vi "UI_(06A)_Set_Stop_State.vi"(3 "error in (no error)":errorcluster, 4 "Settings cluster in":T1={"Defaults"={"Default User"=0.0, "VISA Resource Name "=""}, "Recording and saving"={"Researcher name"="", "Name prefix"="", "Data post-processing"={"Filter type"=enum."Savitzky-Golay", "Length"=31, "Order"=3}, "Stop at"=0.0, "\"Stop at\" enabled"=FALSE, "Default save folder path"=path "", "Acquisition FPS"=enum."Max"}, "Geometry"={"Cage diameter, mm"=0, "Starting angle MIDFIELD"=0, "Starting angle BORDER"=0, "Radius, mm CENTER"=0, "Radius, mm MIDFIELD"=0, "N segments MIDFIELD"=0, "N segments BORDER"=0, "R-gap, mm"=0.0, "Bridge swap"=FALSE, "Bridge H. offset"=0.0, "Bridge V. offset"=0.0, "Twisted neck"=FALSE, "Alt. magn. orientation"=FALSE}, "IO parameters"={"IO general config."=0, "IO 1 configuration"=0, "IO 2 configuration"=0, "IO 3 configuration"=0, "IO 4 configuration"=0, "Activate ext. RS-232"=0, "IO inversion config."=0, "Sync capability"=1}, "Stimulus presets array"=[{"Event type"=0, "Dur., s"=0.0, "Stim., s"=0.0, "TTL out N"=1, "Set/Clear"=FALSE, "Stim. has been set"=FALSE}, {"Event type"=0, "Dur., s"=0.0, "Stim., s"=0.0, "TTL out N"=1, "Set/Clear"=FALSE, "Stim. has been set"=FALSE}, {"Event type"=0, "Dur., s"=0.0, "Stim., s"=0.0, "TTL out N"=1, "Set/Clear"=FALSE, "Stim. has been set"=FALSE}, {"Event type"=0, "Dur., s"=0.0, "Stim., s"=0.0, "TTL out N"=1, "Set/Clear"=FALSE, "Stim. has been set"=FALSE}, {"Event type"=0, "Dur., s"=0.0, "Stim., s"=0.0, "TTL out N"=1, "Set/Clear"=FALSE, "Stim. has been set"=FALSE}, {"Event type"=0, "Dur., s"=0.0, "Stim., s"=0.0, "TTL out N"=1, "Set/Clear"=FALSE, "Stim. has been set"=FALSE}, {"Event type"=0, "Dur., s"=0.0, "Stim., s"=0.0, "TTL out N"=1, "Set/Clear"=FALSE, "Stim. has been set"=FALSE}, {"Event type"=0, "Dur., s"=0.0, "Stim., s"=0.0, "TTL out N"=1, "Set/Clear"=FALSE, "Stim. has been set"=FALSE}, {"Event type"=0, "Dur., s"=0.0, "Stim., s"=0.0, "TTL out N"=1, "Set/Clear"=FALSE, "Stim. has been set"=FALSE}, {"Event type"=0, "Dur., s"=0.0, "Stim., s"=0.0, "TTL out N"=1, "Set/Clear"=FALSE, "Stim. has been set"=FALSE}, {"Event type"=0, "Dur., s"=0.0, "Stim., s"=0.0, "TTL out N"=1, "Set/Clear"=FALSE, "Stim. has been set"=FALSE}, {"Event type"=0, "Dur., s"=0.0, "Stim., s"=0.0, "TTL out N"=1, "Set/Clear"=FALSE, "Stim. has been set"=FALSE}, {"Event type"=0, "Dur., s"=0.0, "Stim., s"=0.0, "TTL out N"=1, "Set/Clear"=FALSE, "Stim. has been set"=FALSE}, {"Event type"=0, "Dur., s"=0.0, "Stim., s"=0.0, "TTL out N"=1, "Set/Clear"=FALSE, "Stim. has been set"=FALSE}], "Calibration parameters"={"Timing calibration sw/hw"=1.0, "True FPS"=80.0, "True frame time, s"=80.0, "Disp. calibration info"=[]}, "Settings loaded OK"=FALSE} {"Calibration parameters"."True frame time, s" format="%.10g"; "Calibration parameters"."Disp. calibration info"."Speed, µl per ms" format="%.3g"; "Calibration parameters"."True FPS" format="%.10g"; "Calibration parameters"."Timing calibration sw/hw" format="%.10g"; "Stimulus presets array"."Event type" items=["Stay for N seconds"]; "Stimulus presets array"."TTL out N" items=["1"=1, "2"=2, "1+2"=3]; "Recording and saving"."Data post-processing"."Order" min=3 max=11 step=2; "Recording and saving"."Data post-processing"."Length" min=5 max=301 step=2; "Geometry"."Cage diameter, mm" scale=0.0..340.0}, 5 "All references in":T11) -> (0 "error out":errorcluster, 1 "Settings cluster out":T1={"Defaults"={"Default User"=0.0, "VISA Resource Name "=""}, "Recording and saving"={"Researcher name"="", "Name prefix"="", "Data post-processing"={"Filter type"=enum."Savitzky-Golay", "Length"=31, "Order"=3}, "Stop at"=0.0, "\"Stop at\" enabled"=FALSE, "Default save folder path"=path "", "Acquisition FPS"=enum."Max"}, "Geometry"={"Cage diameter, mm"=0, "Starting angle MIDFIELD"=0, "Starting angle BORDER"=0, "Radius, mm CENTER"=0, "Radius, mm MIDFIELD"=0, "N segments MIDFIELD"=0, "N segments BORDER"=0, "R-gap, mm"=0.0, "Bridge swap"=FALSE, "Bridge H. offset"=0.0, "Bridge V. offset"=0.0, "Twisted neck"=FALSE, "Alt. magn. orientation"=FALSE}, "IO parameters"={"IO general config."=0, "IO 1 configuration"=0, "IO 2 configuration"=0, "IO 3 configuration"=0, "IO 4 configuration"=0, "Activate ext. RS-232"=0, "IO inversion config."=0, "Sync capability"=1}, "Stimulus presets array"=[{"Event type"=0, "Dur., s"=0.0, "Stim., s"=0.0, "TTL out N"=1, "Set/Clear"=FALSE, "Stim. has been set"=FALSE}, {"Event type"=0, "Dur., s"=0.0, "Stim., s"=0.0, "TTL out N"=1, "Set/Clear"=FALSE, "Stim. has been set"=FALSE}, {"Event type"=0, "Dur., s"=0.0, "Stim., s"=0.0, "TTL out N"=1, "Set/Clear"=FALSE, "Stim. has been set"=FALSE}, {"Event type"=0, "Dur., s"=0.0, "Stim., s"=0.0, "TTL out N"=1, "Set/Clear"=FALSE, "Stim. has been set"=FALSE}, {"Event type"=0, "Dur., s"=0.0, "Stim., s"=0.0, "TTL out N"=1, "Set/Clear"=FALSE, "Stim. has been set"=FALSE}, {"Event type"=0, "Dur., s"=0.0, "Stim., s"=0.0, "TTL out N"=1, "Set/Clear"=FALSE, "Stim. has been set"=FALSE}, {"Event type"=0, "Dur., s"=0.0, "Stim., s"=0.0, "TTL out N"=1, "Set/Clear"=FALSE, "Stim. has been set"=FALSE}, {"Event type"=0, "Dur., s"=0.0, "Stim., s"=0.0, "TTL out N"=1, "Set/Clear"=FALSE, "Stim. has been set"=FALSE}, {"Event type"=0, "Dur., s"=0.0, "Stim., s"=0.0, "TTL out N"=1, "Set/Clear"=FALSE, "Stim. has been set"=FALSE}, {"Event type"=0, "Dur., s"=0.0, "Stim., s"=0.0, "TTL out N"=1, "Set/Clear"=FALSE, "Stim. has been set"=FALSE}, {"Event type"=0, "Dur., s"=0.0, "Stim., s"=0.0, "TTL out N"=1, "Set/Clear"=FALSE, "Stim. has been set"=FALSE}, {"Event type"=0, "Dur., s"=0.0, "Stim., s"=0.0, "TTL out N"=1, "Set/Clear"=FALSE, "Stim. has been set"=FALSE}, {"Event type"=0, "Dur., s"=0.0, "Stim., s"=0.0, "TTL out N"=1, "Set/Clear"=FALSE, "Stim. has been set"=FALSE}, {"Event type"=0, "Dur., s"=0.0, "Stim., s"=0.0, "TTL out N"=1, "Set/Clear"=FALSE, "Stim. has been set"=FALSE}], "Calibration parameters"={"Timing calibration sw/hw"=1.0, "True FPS"=80.0, "True frame time, s"=80.0, "Disp. calibration info"=[]}, "Settings loaded OK"=FALSE} {"Calibration parameters"."True frame time, s" format="%.10g"; "Calibration parameters"."Disp. calibration info"."Speed, µl per ms" format="%.3g"; "Calibration parameters"."True FPS" format="%.10g"; "Calibration parameters"."Timing calibration sw/hw" format="%.10g"; "Stimulus presets array"."Event type" items=["Stay for N seconds"]; "Stimulus presets array"."TTL out N" items=["1"=1, "2"=2, "1+2"=3]; "Recording and saving"."Data post-processing"."Order" min=3 max=11 step=2; "Recording and saving"."Data post-processing"."Length" min=5 max=301 step=2; "Geometry"."Cage diameter, mm" scale=0.0..340.0}, 2 "All references out":T11)   [LabVIEW 2018, in "Tracker.lvlib"]
uses:
  Tracker.lvlib
  Controls/CTL_All_References.ctl
  Controls/CTL_Controls_References.ctl
  Controls/CTL_Indicators_References.ctl
  Controls/CTL_Panes_and_VIs_References.ctl
  Controls/CTL_Histogram_Properties.ctl
  <vilib>/Utility/miscctls.llb/LVRangeTypeDef.ctl
  Controls/CTL_Settings_cluster.ctl
  Controls/CTL_Filter_selector.ctl
  Controls/CTL_Acquisition_speed_selector.ctl
  Controls/CTL_Segmented_plot_parameters.ctl
  Controls/CTL_IO_params_cluster.ctl
  Controls/CTL_Single_stimulus_setting.ctl
  Controls/CTL_Calibration_parameters.ctl
  Controls/CTL_Dispenser_calibration_info.ctl
  <vilib>/Utility/error.llb/Error Cluster From Error Code.vi
  <vilib>/ErrorRing/Error Ring.xnode
panel:
  in  "Histogram initialization cluster":T9={"X Scale.Range"={"Minimum"=0.0, "Maximum"=13.0, "Increment"=1.0, "Minor Increment"=1.0, "Start"=0.0}, "Caption.Text"="Zone preference (normalized)", "X Scale.Offset and Multiplier:Multiplier"=1.0, "X Scale.Offset and Multiplier:Offset"=0.0, "X Scale.Scale Fit"=2, "X Scale.Display Format:Precision"=0, "Y Scale.Mapping Mode"=0, "Zones preference empty initialized array"=[0, 0, 0, 0, 0, 0, 0, 0, 0, 0, 0, 0, 0, 0], "Plot.Fill/Point Color"=15790320}
  out "Panes references":T14
  out "Controls references params":string[][](array[string])
  out "Indicators references params":string[][](array[string])
  out "Indicators references":T13
  out "Controls references":T12
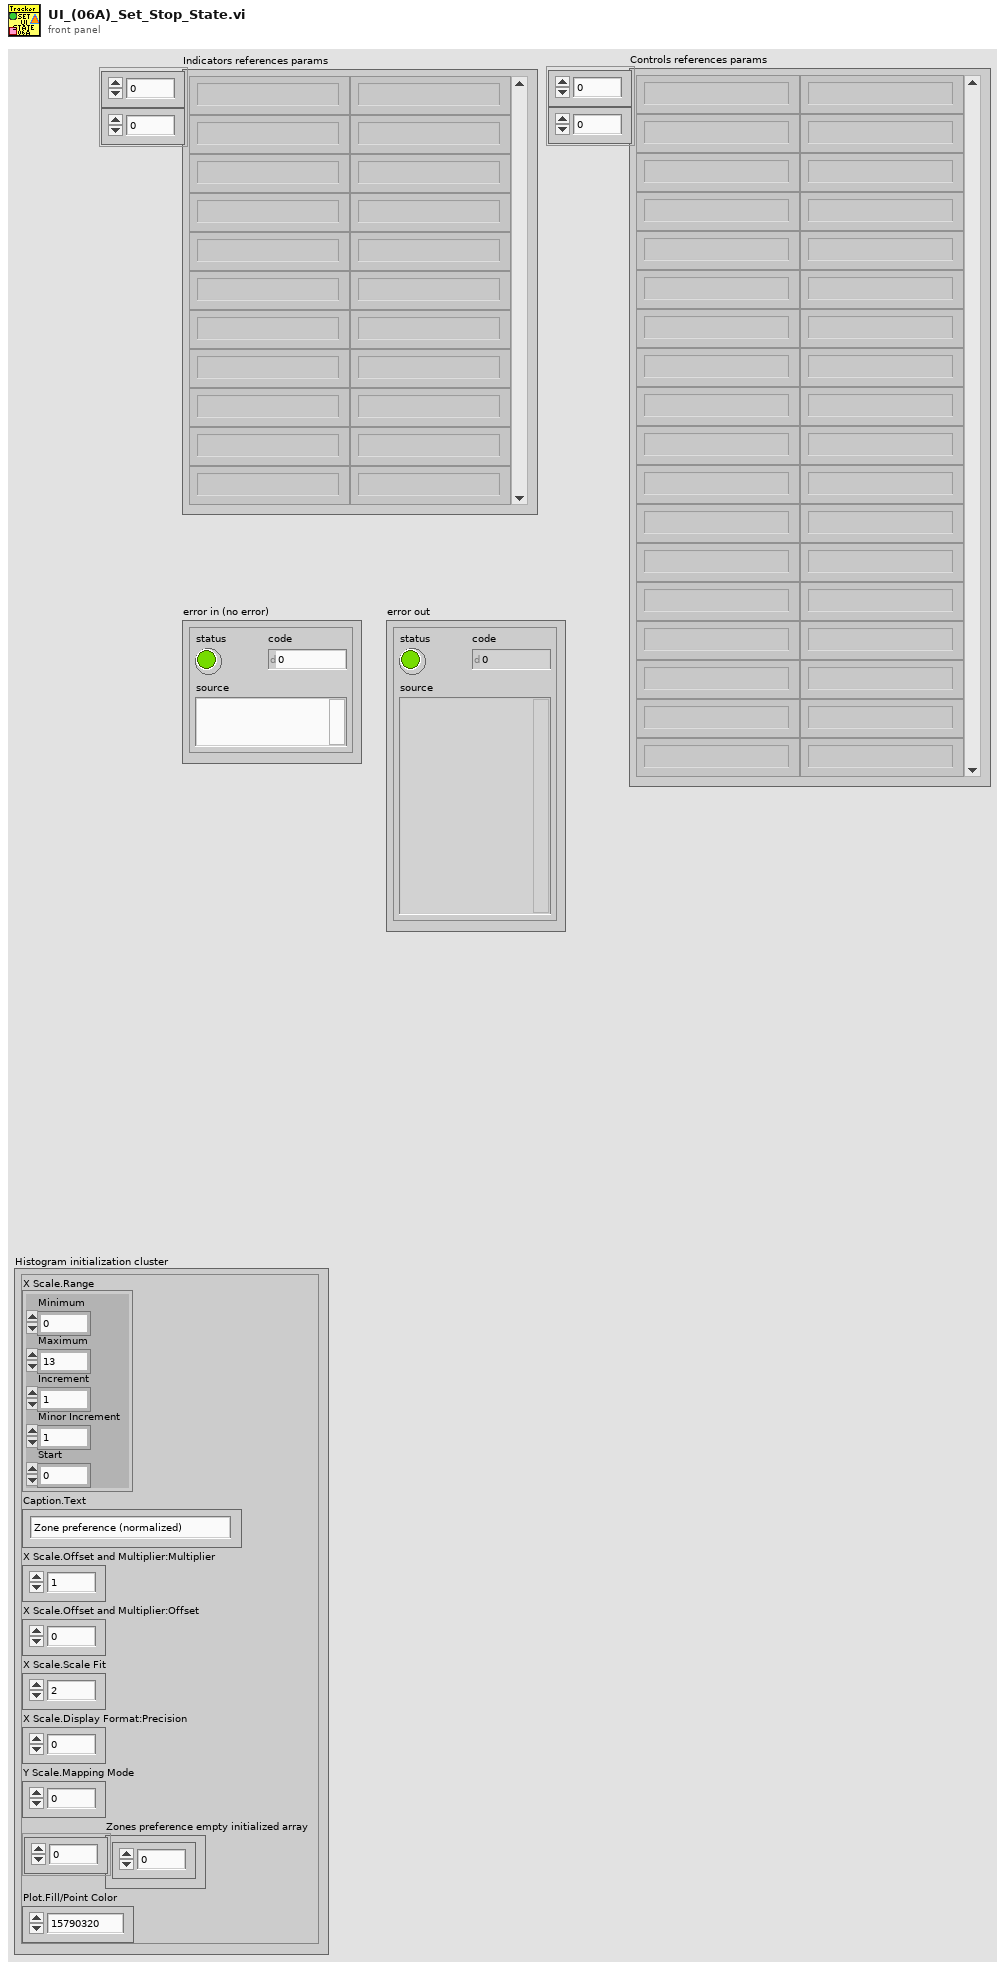
[diagram p1: front panel]
types:
  T1 = typedef "Tracker.lvlib/CTL_Settings_cluster.ctl" = cluster{"Defaults":cluster{"Default User":dbl, "VISA Resource Name ":string}, "Recording and saving":cluster{"Researcher name":string, "Name prefix":string, "Data post-processing":T2, "Stop at":dbl, "\"Stop at\" enabled":bool, "Default save folder path":path, "Acquisition FPS":T3}, "Geometry":T4, "IO parameters":T5, "Stimulus presets array":T6[], "Calibration parameters":T7, "Settings loaded OK":bool}
  T2 = typedef "Tracker.lvlib/CTL_Filter_selector.ctl" = cluster{"Filter type":enum16{"None", "Savitzky-Golay"}, "Length":i32, "Order":i32}
  T3 = typedef "Tracker.lvlib/CTL_Acquisition_speed_selector.ctl" = enum16{"Max", "Optimal", "Eco"}
  T4 = typedef "Tracker.lvlib/CTL_Segmented_plot_parameters.ctl" = cluster{"Cage diameter, mm":u16, "Starting angle MIDFIELD":i16, "Starting angle BORDER":i16, "Radius, mm CENTER":u16, "Radius, mm MIDFIELD":u16, "N segments MIDFIELD":u8, "N segments BORDER":u8, "R-gap, mm":sgl, "Bridge swap":bool, "Bridge H. offset":sgl, "Bridge V. offset":sgl, "Twisted neck":bool, "Alt. magn. orientation":bool}
  T5 = typedef "Tracker.lvlib/CTL_IO_params_cluster.ctl" = cluster{"IO general config.":u16, "IO 1 configuration":u16, "IO 2 configuration":u16, "IO 3 configuration":u16, "IO 4 configuration":u16, "Activate ext. RS-232":u16, "IO inversion config.":u16, "Sync capability":u8}
  T6 = typedef "Tracker.lvlib/CTL_Single_stimulus_setting.ctl" = cluster{"Event type":u16, "Dur., s":sgl, "Stim., s":sgl, "TTL out N":u16, "Set/Clear":bool, "Stim. has been set":bool}
  T7 = typedef "Tracker.lvlib/CTL_Calibration_parameters.ctl" = cluster{"Timing calibration sw/hw":dbl, "True FPS":dbl, "True frame time, s":dbl, "Disp. calibration info":T8}
  T8 = typedef "Tracker.lvlib/CTL_Dispenser_calibration_info.ctl" = cluster{"Channel":u8, "Speed, µl per ms":dbl}[]
  T9 = typedef "Tracker.lvlib/CTL_Histogram_Properties.ctl" = cluster{"X Scale.Range":T10, "Caption.Text":string, "X Scale.Offset and Multiplier:Multiplier":dbl, "X Scale.Offset and Multiplier:Offset":dbl, "X Scale.Scale Fit":u8, "X Scale.Display Format:Precision":u8, "Y Scale.Mapping Mode":u8, "Zones preference empty initialized array":i32[], "Plot.Fill/Point Color":u32}
  T10 = typedef "LVRangeTypeDef.ctl" = cluster{"Minimum":dbl, "Maximum":dbl, "Increment":dbl, "Minor Increment":dbl, "Start":dbl}
  T11 = typedef "Tracker.lvlib/CTL_All_References.ctl" = cluster{"Controls references":T12, "Indicators references":T13, "Service references":T14}
  T12 = typedef "Tracker.lvlib/CTL_Controls_References.ctl" = cluster{"Check HW connection":refnum<vi>, "Start Tracking button":refnum<vi>, "Reset zones":refnum<vi>, "Reset stimuli":refnum<vi>, "Record/Stop":refnum<vi>, "Reset barplot":refnum<vi>, "Multiplyer of chart RX":refnum<vi>, "Show zones":refnum<vi>, "Show magnets":refnum<vi>, "Show heatmap":refnum<vi>, "Show full track":refnum<vi>, "Open File":refnum<vi>, "Play/Pause":refnum<vi>, "Trace, s":refnum<vi>, "Playback speed":refnum<vi>, "Timeline":refnum<vi>, "By Zone stim. setup":refnum<vi>, "Set, Rec and Analyse Tab":refnum<vi>, "Cage radial segmentation":refnum<vi>, "Set IO config":refnum<vi>, "Rainbow (time)":refnum<vi>, "Rainbow (speed)":refnum<vi>}
  T13 = typedef "Tracker.lvlib/CTL_Indicators_References.ctl" = cluster{"HW info":refnum<vi>, "Port":refnum<vi>, "Ready":refnum<vi>, "IO status indicator":refnum<vi>, "Current Time":refnum<vi>, "Record timestamp":refnum<vi>, "Mouse speed":refnum<vi>, "Mouse speed, mm/s":refnum<vi>, "Running, perc. of time":refnum<vi>, "Histograms":refnum<vi>, "Cage size":refnum<vi>}
  T14 = typedef "Tracker.lvlib/CTL_Panes_and_VIs_References.ctl" = cluster{"Pane":refnum<vi>, "This VI":refnum<vi>, "Menu":refnum<k9>}
  T15 = enum8{"Enabled", "Disabled", "Disabled and Grayed Out"}
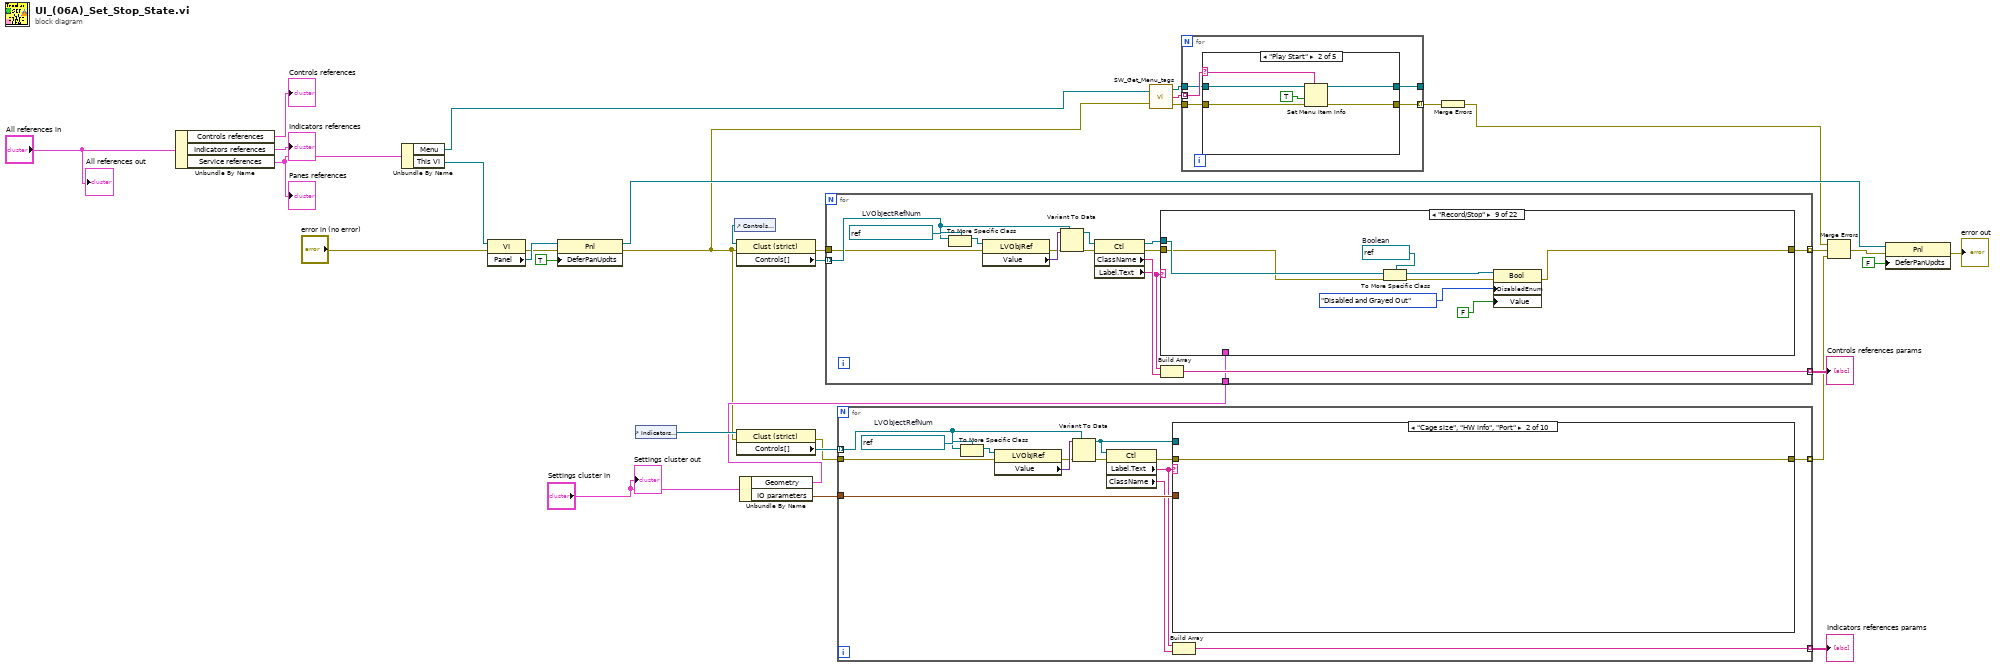
[diagram p0: block diagram]
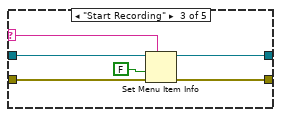
[diagram p3: hidden frame]
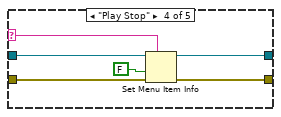
[diagram p4: hidden frame]
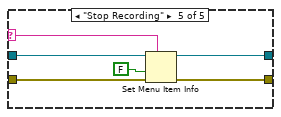
[diagram p5: hidden frame]
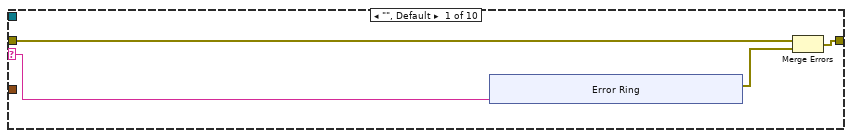
[diagram p6: hidden frame]
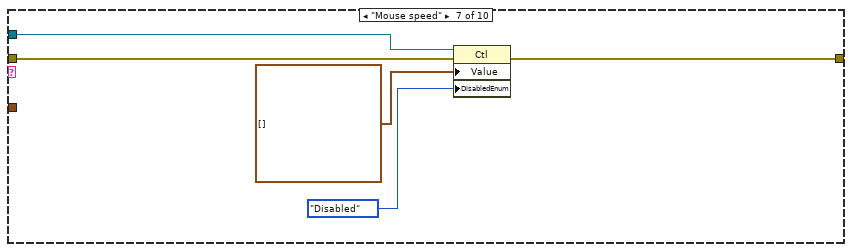
[diagram p11: hidden frame]
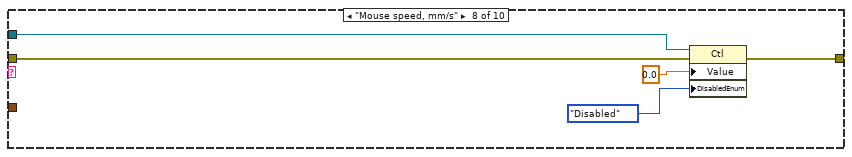
[diagram p12: hidden frame]
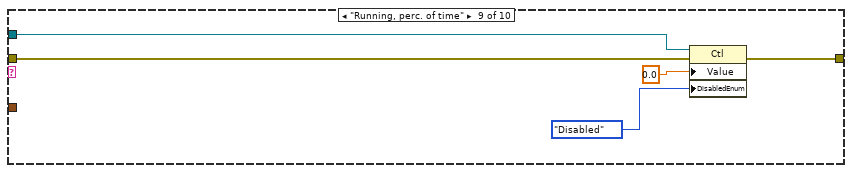
[diagram p13: hidden frame]
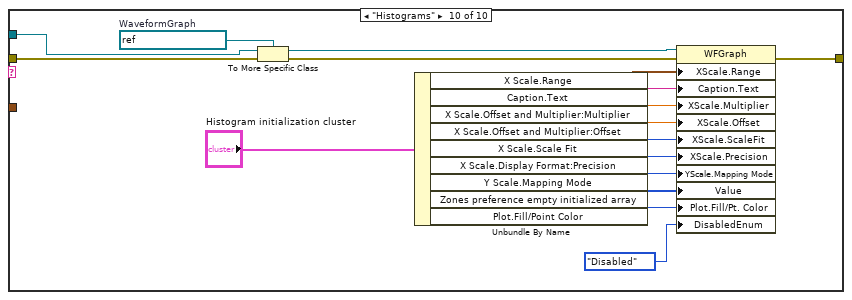
[diagram p14: hidden frame]
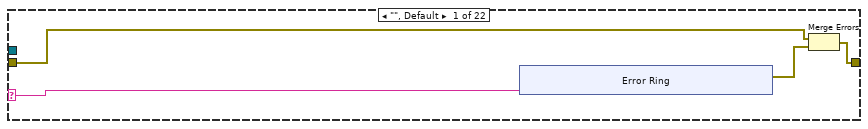
[diagram p15: hidden frame]
diagram:
  n1 = Unbundle By Name("All references in") -> ("Controls references"=→"Controls references":T12, "Indicators references"=→"Indicators references":T13, "Service references"=w24:T14)
  "Panes references" <- w24
  n2 = Unbundle By Name(w24) -> ("Menu"=w3:refnum<k9>, "This VI"=w21:refnum<vi>)
  n3 = property class="VI"(reference=w21, error in="error in (no error)") -> (error out=w14:errorcluster, "Panel"=w23:refnum<vi>)  [unwired: 1 out]
  n4 = property class="Pnl"(reference=w23, error in=w14, "DeferPanUpdts"=TRUE ("Defer Panel Updates")) -> (reference out=w15:refnum<vi>, error out=w2:errorcluster)
  n5 = control-ref of="Indicators references"() -> (w27:refnum<vi>)
  n6 = control-ref of="Controls references"() -> (w29:refnum<vi>)
  n7 = property class="Clust (strict)"(reference=w29, error in=w2) -> (error out=w20:errorcluster, "Controls[]"=w30:refnum<vi>[])  [unwired: 1 out]
  n8 = property class="Clust (strict)"(reference=w27, error in=w2) -> (error out=w19:errorcluster, "Controls[]"=w28:refnum<vi>[])  [unwired: 1 out]
  n9 = Unbundle By Name("Settings cluster in") -> ("Geometry"=w8:T4, "IO parameters"=w10:T5)
  n10 = for {
    tunnel: w30 -> [w45] mode=indexing
    tunnel: [w42] -> w25 mode=indexing
    tunnel: w20 -> [w41]
    tunnel: [w37] -> w12 mode=indexing
    tunnel: w8 -> [w34]
    w47 = refnum<vi> refnum  # LVObjectRefNum
    n11 = To More Specific Class(target class=w47, reference=w45) -> (specific class reference=w48:refnum<vi>)  [unwired: 1 in, 1 out]
    n12 = property class="LVObjRef"(reference=w48, error in=w41) -> (error out=w40:errorcluster, "Value"=w46:variant)  [unwired: 1 out]
    n13 = Variant To Data(error in=w40, type=w45, Variant=w46) -> (data=w44:refnum<vi>, error out=w39:errorcluster)
    n14 = property class="Ctl"(reference=w44, error in=w39) -> (reference out=w35:refnum<vi>, error out=w36:errorcluster, "ClassName"=w43:string, "Label.Text"=w38:string)
    n15 = case shown="\"Record/Stop\"" w38 {
      selector: w38 -> [w49 _ _ _ _ _ _ _ _ _ _ _ _ _ _ _ _ _ _ _ _ _]
      tunnel: [w51 w60 w61 w62 w63 w64 w65 w66 w67 w77 w85 w93 w99 w100 w109 w117 w123 w125 w134 w142 w150 w156] -> w37
      tunnel: w36 -> [w52 w60 w61 w62 w63 w64 w65 w66 w68 w79 w87 w95 w99 w102 w111 w119 w123 w126 w136 w144 w152 w156]
      tunnel: w35 -> [_ _ _ _ _ _ _ _ w69 w82 w90 w98 _ w101 w114 w122 _ w127 w139 w147 w155 _]
      tunnel: w34 -> [_ _ _ _ _ _ _ _ _ _ _ _ _ _ _ _ _ _ _ _ _ _]
      frame "", Default {
        n16 = xnode "Error Ring"("parameter 0"=w49) -> ("error out"=w50:errorcluster)
        n17 = Merge Errors(w52, w50) -> (w51:errorcluster)
      }
      frame "Cage radial segmentation" {
      }
      frame "Set/Rec and Analyse Tab" {
      }
      frame "Check HW connection" {
      }
      frame "Save settings" {
      }
      frame "Set IO config" {
      }
      frame "Reset zones" {
      }
      frame "Reset stimuli" {
      }
      frame "Record/Stop" {
        w70 = refnum<vi> refnum  # Boolean
        n18 = To More Specific Class(target class=w70, reference=w69, error in=w68) -> (specific class reference=w74:refnum<vi>, error out=w73:errorcluster)
        n19 = property class="Bool"(reference=w74, error in=w73, "DisabledEnum"=T15."Disabled and Grayed Out" ("Disabled"), "Value"=FALSE) -> (error out=w67:errorcluster)  [unwired: 1 out]
      }
      frame "Reset barplot" {
        w81 = refnum<vi> refnum  # Boolean
        n20 = To More Specific Class(target class=w81, reference=w82, error in=w79) -> (specific class reference=w80:refnum<vi>, error out=w78:errorcluster)
        n21 = property class="Bool"(reference=w80, error in=w78, "Value"=FALSE, "DisabledEnum"=T15."Enabled" ("Disabled")) -> (error out=w77:errorcluster)  [unwired: 1 out]
      }
      frame "Multiplyer of chart RX" {
        w89 = refnum<vi> refnum  # Slide
        n22 = To More Specific Class(target class=w89, reference=w90, error in=w87) -> (specific class reference=w88:refnum<vi>, error out=w86:errorcluster)
        n23 = property class="Slide"(reference=w88, error in=w86, "Value"=u8 1, "DisabledEnum"=T15."Enabled" ("Disabled")) -> (error out=w85:errorcluster)  [unwired: 1 out]
      }
      frame "Show zones" {
        w97 = refnum<vi> refnum  # Boolean
        n24 = To More Specific Class(target class=w97, reference=w98, error in=w95) -> (specific class reference=w96:refnum<vi>, error out=w94:errorcluster)
        n25 = property class="Bool"(reference=w96, error in=w94, "Value"=TRUE, "DisabledEnum"=T15."Enabled" ("Disabled")) -> (error out=w93:errorcluster)  [unwired: 1 out]
      }
      frame "Show magnets" {
      }
      frame "Rainbow (speed)", "Rainbow (time)" {
        w103 = refnum<vi> refnum  # Boolean
        n26 = To More Specific Class(target class=w103, reference=w101, error in=w102) -> (specific class reference=w105:refnum<vi>, error out=w106:errorcluster)
        n27 = property class="Bool"(reference=w105, error in=w106, "DisabledEnum"=T15."Enabled" ("Disabled")) -> (error out=w100:errorcluster)  [unwired: 1 out]
      }
      frame "Show heatmap" {
        w113 = refnum<vi> refnum  # Boolean
        n28 = To More Specific Class(target class=w113, reference=w114, error in=w111) -> (specific class reference=w112:refnum<vi>, error out=w110:errorcluster)
        n29 = property class="Bool"(reference=w112, error in=w110, "Value"=FALSE, "DisabledEnum"=T15."Disabled and Grayed Out" ("Disabled")) -> (error out=w109:errorcluster)  [unwired: 1 out]
      }
      frame "Show full track" {
        w121 = refnum<vi> refnum  # Boolean
        n30 = To More Specific Class(target class=w121, reference=w122, error in=w119) -> (specific class reference=w120:refnum<vi>, error out=w118:errorcluster)
        n31 = property class="Bool"(reference=w120, error in=w118, "Value"=FALSE, "DisabledEnum"=T15."Disabled and Grayed Out" ("Disabled")) -> (error out=w117:errorcluster)  [unwired: 1 out]
      }
      frame "Open File" {
      }
      frame "Play/Pause" {
        w128 = refnum<vi> refnum  # Boolean
        n32 = To More Specific Class(target class=w128, reference=w127, error in=w126) -> (specific class reference=w131:refnum<vi>, error out=w130:errorcluster)
        n33 = property class="Bool"(reference=w131, error in=w130, "DisabledEnum"=T15."Enabled" ("Disabled"), "Value"=FALSE) -> (error out=w125:errorcluster)  [unwired: 1 out]
      }
      frame "Trace, s" {
        w138 = refnum<vi> refnum  # Slide
        n34 = To More Specific Class(target class=w138, reference=w139, error in=w136) -> (specific class reference=w137:refnum<vi>, error out=w135:errorcluster)
        n35 = property class="Slide"(reference=w137, error in=w135, "Value"=u8 5, "DisabledEnum"=T15."Enabled" ("Disabled")) -> (error out=w134:errorcluster)  [unwired: 1 out]
      }
      frame "Playback speed" {
        w146 = refnum<vi> refnum  # Ring
        n36 = To More Specific Class(target class=w146, reference=w147, error in=w144) -> (specific class reference=w145:refnum<vi>, error out=w143:errorcluster)
        n37 = property class="Ring"(reference=w145, error in=w143, "Value"=u8 3, "DisabledEnum"=T15."Disabled and Grayed Out" ("Disabled")) -> (error out=w142:errorcluster)  [unwired: 1 out]
      }
      frame "Timeline" {
        w154 = refnum<vi> refnum  # Slide
        n38 = To More Specific Class(target class=w154, reference=w155, error in=w152) -> (specific class reference=w153:refnum<vi>, error out=w151:errorcluster)
        n39 = property class="Slide"(reference=w153, error in=w151, "Value"=u8 5, "DisabledEnum"=T15."Disabled and Grayed Out" ("Disabled")) -> (error out=w150:errorcluster)  [unwired: 1 out]
      }
      frame "By Zone stim. setup" {
      }
    }
    n40 = Build Array(w38, w43) -> (w42:string[])
  }
  "Controls references params" <- w25
  n41 = for {
    tunnel: w28 -> [w167] mode=indexing
    tunnel: [w157] -> w26 mode=indexing
    tunnel: w19 -> [w165]
    tunnel: [w161] -> w18 mode=indexing
    tunnel: w10 -> [w160]
    w169 = refnum<vi> refnum  # LVObjectRefNum
    n42 = To More Specific Class(target class=w169, reference=w167) -> (specific class reference=w170:refnum<vi>)  [unwired: 1 in, 1 out]
    n43 = property class="LVObjRef"(reference=w170, error in=w165) -> (error out=w164:errorcluster, "Value"=w168:variant)  [unwired: 1 out]
    n44 = Variant To Data(error in=w164, type=w167, Variant=w168) -> (data=w166:refnum<vi>, error out=w163:errorcluster)
    n45 = property class="Ctl"(reference=w166, error in=w163) -> (error out=w162:errorcluster, "Label.Text"=w159:string, "ClassName"=w158:string)  [unwired: 1 out]
    n46 = case shown="\"Cage size\", \"HW info\", \"Port\"" w159 {
      selector: w159 -> [w171 _ _ _ _ _ _ _ _ _]
      tunnel: w166 -> [_ _ _ _ _ _ w191 w196 w201 w218]
      tunnel: w162 -> [w174 w182 w183 w184 w185 w186 w190 w195 w200 w204]
      tunnel: [w173 w182 w183 w184 w185 w186 w189 w194 w199 w217] -> w161
      tunnel: w160 -> [_ _ _ _ _ _ _ _ _ _]
      frame "", Default {
        n47 = xnode "Error Ring"("parameter 0"=w171) -> ("error out"=w172:errorcluster)
        n48 = Merge Errors(w174, w172) -> (w173:errorcluster)
      }
      frame "Cage size", "HW info", "Port" {
      }
      frame "Ready" {
      }
      frame "IO status indicator" {
      }
      frame "Current Time" {
      }
      frame "Record timestamp" {
      }
      frame "Mouse speed" {
        n49 = property class="Ctl"(reference=w191, error in=w190, "Value"=waveform(dbl)[] [] ("History Data"), "DisabledEnum"=T15."Disabled" ("Disabled")) -> (error out=w189:errorcluster)  [unwired: 1 out]
      }
      frame "Mouse speed, mm/s" {
        n50 = property class="Ctl"(reference=w196, error in=w195, "Value"=0.0, "DisabledEnum"=T15."Disabled" ("Disabled")) -> (error out=w194:errorcluster)  [unwired: 1 out]
      }
      frame "Running, perc. of time" {
        n51 = property class="Ctl"(reference=w201, error in=w200, "Value"=0.0, "DisabledEnum"=T15."Disabled" ("Disabled")) -> (error out=w199:errorcluster)  [unwired: 1 out]
      }
      frame "Histograms" {
        w215 = refnum<vi> refnum  # WaveformGraph
        n52 = To More Specific Class(target class=w215, reference=w218, error in=w204) -> (specific class reference=w216:refnum<vi>, error out=w203:errorcluster)
        n53 = Unbundle By Name("Histogram initialization cluster") -> ("X Scale.Range"=w213:T10, "Caption.Text"=w212:string, "X Scale.Offset and Multiplier:Multiplier"=w211:dbl, "X Scale.Offset and Multiplier:Offset"=w210:dbl, "X Scale.Scale Fit"=w209:u8, "X Scale.Display Format:Precision"=w208:u8, "Y Scale.Mapping Mode"=w207:u8, "Zones preference empty initialized array"=w206:i32[], "Plot.Fill/Point Color"=w205:u32)
        n54 = property class="WFGraph"(reference=w216, error in=w203, "XScale.Range"=w213, "Caption.Text"=w212, "XScale.Multiplier"=w211, "XScale.Offset"=w210, "XScale.ScaleFit"=w209, "XScale.Precision"=w208, "YScale.Mapping Mode"=w207, "Value"=w206, "Plot.Fill/Pt. Color"=w205, "DisabledEnum"=T15."Disabled" ("Disabled")) -> (error out=w217:errorcluster)  [unwired: 1 out]
      }
    }
    n55 = Build Array(w159, w158) -> (w157:string[])
  }
  "Indicators references params" <- w26
  n56 = call "SW_Get_Menu_tags.vi"("Menu ref in"=w3, "error in (no error)"=w2) -> ("Menu ref out"=w5:refnum<k9>, "(Sub)menu tags"=w7:string[], "error out"=w6:errorcluster)
  n57 = for {
    tunnel: w7 -> [w223] mode=indexing
    tunnel: w6 -> [w222]
    tunnel: [w221] -> w4 mode=indexing
    tunnel: [w220] -> _
    tunnel: w5 -> [w219]
    n58 = case shown="\"Play Start\"" w223 {
      selector: w223 -> [_ w231 w237 w243 w249]
      tunnel: w222 -> [w225 w229 w235 w241 w247]
      tunnel: [w225 w228 w234 w240 w246] -> w221
      tunnel: [w224 w227 w233 w239 w245] -> w220
      tunnel: w219 -> [w224 w226 w232 w238 w244]
      frame "", Default {
      }
      frame "Play Start" {
        n59 = Set Menu Item Info(7:w231, 8:w229, 9:TRUE ("enabled"), 11:w226) -> (0:w228:errorcluster, 3:w227:refnum<k9>)  [unwired: 3 in]
      }
      frame "Start Recording" {
        n60 = Set Menu Item Info(7:w237, 8:w235, 9:FALSE ("enabled"), 11:w232) -> (0:w234:errorcluster, 3:w233:refnum<k9>)  [unwired: 3 in]
      }
      frame "Play Stop" {
        n61 = Set Menu Item Info(7:w243, 8:w241, 9:FALSE ("enabled"), 11:w238) -> (0:w240:errorcluster, 3:w239:refnum<k9>)  [unwired: 3 in]
      }
      frame "Stop Recording" {
        n62 = Set Menu Item Info(7:w249, 8:w247, 9:FALSE ("enabled"), 11:w244) -> (0:w246:errorcluster, 3:w245:refnum<k9>)  [unwired: 3 in]
      }
    }
  }
  n63 = Merge Errors(w4) -> (w1:errorcluster)
  n64 = Merge Errors(w1, w12, w18) -> (w17:errorcluster)
  n65 = property class="Pnl"(reference=w15, error in=w17, "DeferPanUpdts"=FALSE ("Defer Panel Updates")) -> (error out=→"error out":errorcluster)  [unwired: 1 out]
  "All references out" <- "All references in"
  "Settings cluster out" <- "Settings cluster in"
